vi "Send CALL.vi"(0 "WAMP Client in":refnum<class "WAMP Client.lvclass">, 5 "Call Request":T7, 9 "Message Loop Shift Register Data":T1, 11 "error in (no error)":errorcluster) -> (4 "WAMP Client out":refnum<class "WAMP Client.lvclass">, 10 "Message Loop Shift Register Data (out)":T1, 15 "error out":errorcluster)   [LabVIEW 2021, in "wamplv.lvlib" / "WAMP Client.lvclass"]
uses:
  WAMP Client.lvclass
  TypeDef/CALL Request Data.ctl
  API/TypeDefs/RESULT payload.ctl
  API/TypeDefs/Combined error.ctl
  API/TypeDefs/WAMP error.ctl
  TypeDef/Message Loop Shift Reg Data.ctl
  TypeDef/REGISTER Request Data.ctl
  TypeDef/Success or error.ctl
  TypeDef/Publish Requests Map.ctl
  TypeDef/PUBLISH Request Data.ctl
  TypeDef/PUBLISH result.ctl
  TypeDef/Endpoint Data.ctl
  TypeDef/CALL Request Map.ctl
  TypeDef/SUBSCRIBE Requests Map.ctl
  TypeDef/SUBSCRIBE Request Data.ctl
  TypeDef/Subscribe Result.ctl
  TypeDef/EVENT payload.ctl
  TypeDef/Subscriptions Map.ctl
  TypeDef/Subscription Details.ctl
  TypeDef/Unsubscribe Requests Map.ctl
  TypeDef/UNSUBSCRIBE Request Data.ctl
  TypeDef/UNSUBSCRIBE Result.ctl
  TypeDef/Unregister requests map.ctl
  TypeDef/Unregister request.ctl
  TypeDef/WAMP Message Codes.ctl
  WAMP Client.lvclass/WAMP Client.ctl
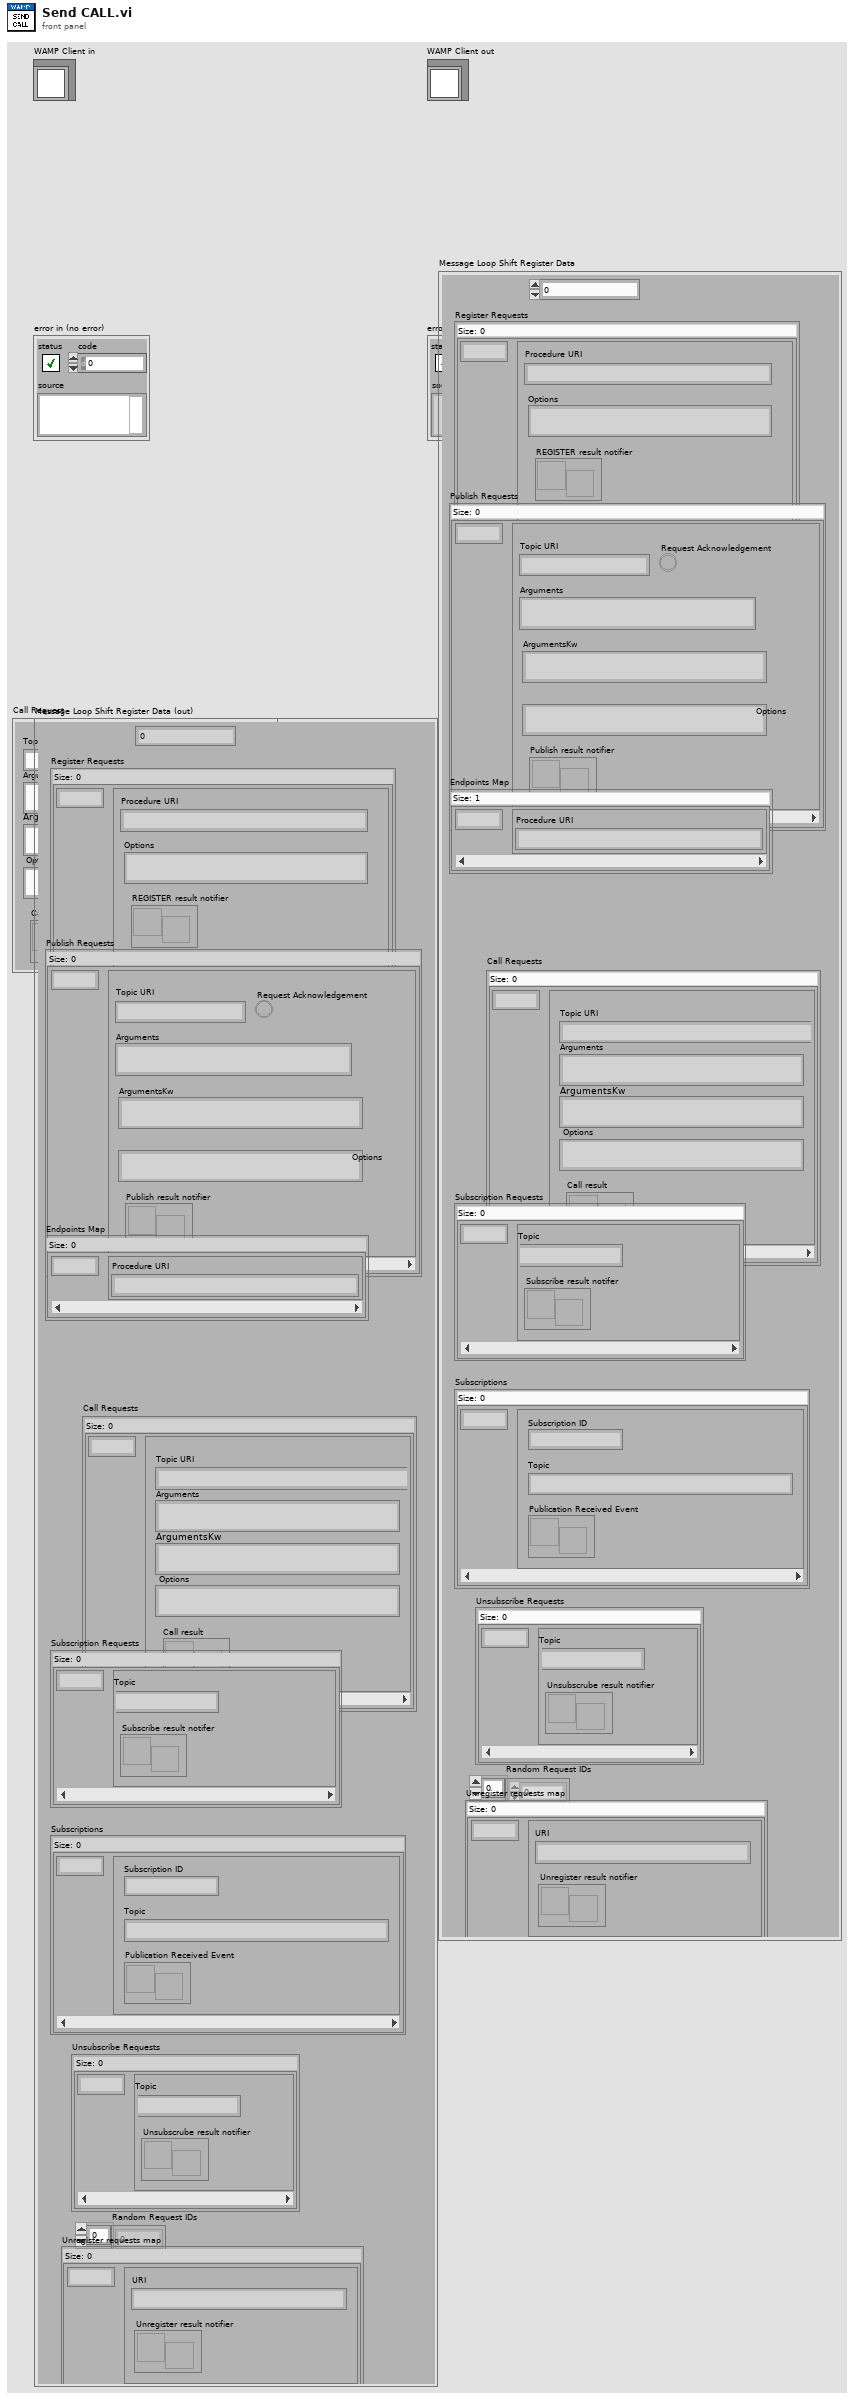
[diagram p1: front panel]
types:
  T1 = typedef "wamplv.lvlib/WAMP Client.lvclass/Message Loop Shift Reg Data.ctl" = cluster{"Last Request ID":u64, "Register Requests":map{u64, T2}, "Publish Requests":T3, "Endpoints Map":map{u64, T5}, "Call Requests":T6, "Subscription Requests":T8, "Subscriptions":T10, "Unsubscribe Requests":T12, "Random Request IDs":u64[], "Unregister requests map":T14}
  T2 = typedef "wamplv.lvlib/WAMP Client.lvclass/REGISTER Request Data.ctl" = cluster{"Procedure URI":string, "Options":string, "REGISTER result notifier":refnum<notifier>}
  T3 = typedef "wamplv.lvlib/WAMP Client.lvclass/Publish Requests Map.ctl" = map{u64, T4}
  T4 = typedef "wamplv.lvlib/WAMP Client.lvclass/PUBLISH Request Data.ctl" = cluster{"Topic URI":string, "Arguments":string, "ArgumentsKw":string, "Request Acknowledgement":bool, "Options":string, "Publish result notifier":refnum<notifier>}
  T5 = typedef "wamplv.lvlib/WAMP Client.lvclass/Endpoint Data.ctl" = cluster{"Procedure URI":string}
  T6 = typedef "wamplv.lvlib/WAMP Client.lvclass/CALL Request Map.ctl" = map{u64, T7}
  T7 = typedef "wamplv.lvlib/WAMP Client.lvclass/CALL Request Data.ctl" = cluster{"Topic URI":string, "Arguments":string, "ArgumentsKw":string, "Options":string, "Call result":refnum<notifier>}
  T8 = typedef "wamplv.lvlib/WAMP Client.lvclass/SUBSCRIBE Requests Map.ctl" = map{u64, T9}
  T9 = typedef "wamplv.lvlib/WAMP Client.lvclass/SUBSCRIBE Request Data.ctl" = cluster{"Topic":string, "Subscribe result notifer":refnum<notifier>}
  T10 = typedef "wamplv.lvlib/WAMP Client.lvclass/Subscriptions Map.ctl" = map{u64, T11}
  T11 = typedef "wamplv.lvlib/WAMP Client.lvclass/Subscription Details.ctl" = cluster{"Subscription ID":u64, "Topic":string, "Publication Received Event":refnum<user-event>}
  T12 = typedef "wamplv.lvlib/WAMP Client.lvclass/Unsubscribe Requests Map.ctl" = map{u64, T13}
  T13 = typedef "wamplv.lvlib/WAMP Client.lvclass/UNSUBSCRIBE Request Data.ctl" = cluster{"Topic":string, "Unsubscrube result notifier":refnum<notifier>}
  T14 = typedef "wamplv.lvlib/WAMP Client.lvclass/Unregister requests map.ctl" = map{u64, T15}
  T15 = typedef "wamplv.lvlib/WAMP Client.lvclass/Unregister request.ctl" = cluster{"URI":string, "Unregister result notifier":refnum<notifier>}
  T16 = typedef "wamplv.lvlib/WAMP Client.lvclass/WAMP Message Codes.ctl" = u16
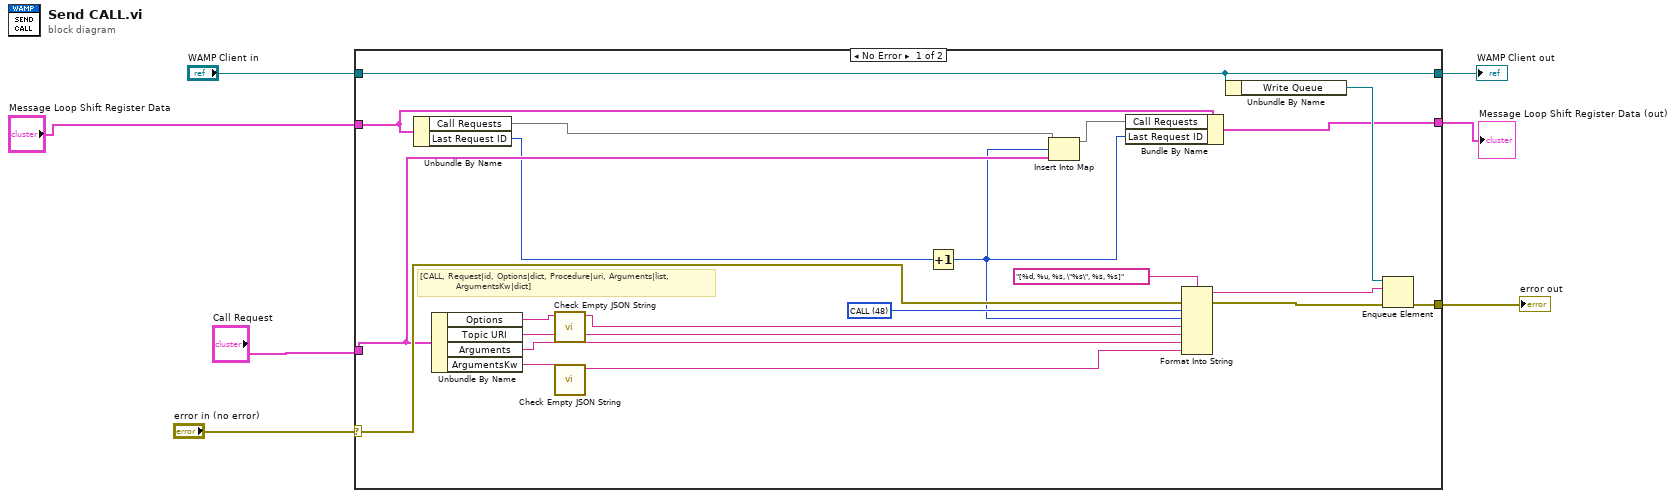
[diagram p0: block diagram]
diagram:
  n1 = case shown="No Error" "error in (no error)" {
    selector: "error in (no error)" -> [w23 w31]
    tunnel: [w28 w31] -> w6
    tunnel: [w22 w30] -> w4
    tunnel: "WAMP Client in" -> [w22 w30]
    tunnel: "Call Request" -> [w18 _]
    tunnel: "Message Loop Shift Register Data" -> [w15 w29]
    tunnel: [w14 w29] -> w1
    frame No Error {
      w20 = T16 48 items=["HELLO"=1, "WELCOME"=2, "ABORT"=3, "GOODBYE"=6, "ERROR"=8, "PUBLISH"=16, "PUBLISHED"=17, "SUBSCRIBE"=32, "SUBSCRIBED"=33, "UNSUBSCRIBE"=34, "UNSUBSCRIBED"=35, "EVENT"=36, "CALL"=48, "RESULT"=59, "REGISTER"=64, "REGISTERED"=65, "UNREGISTER"=66, "UNREGISTERED"=67, "INVOCATION"=68, "YIELD"=70] ("Message Codes")
      # "[CALL, Request|id, Options|dict, Procedure|uri, Arguments|list,\n            ArgumentsKw|dict]"
      n2 = Unbundle By Name(w15) -> ("Call Requests"=w17:T6, "Last Request ID"=w13:u64)
      n3 = Unbundle By Name(w18) -> ("Options"=w9:string, "Topic URI"=w19:string, "Arguments"=w21:string, "ArgumentsKw"=w11:string)
      n4 = call "Check Empty JSON String.vi"("JSON"=w9) -> ("JSON"=w8:string)  [unwired: 10 in]
      n5 = call "Check Empty JSON String.vi"("JSON"=w11) -> ("JSON"=w10:string)  [unwired: 10 in]
      n6 = Increment(x=w13) -> (x+1=w12:u64)
      n7 = Insert Into Map(map in=w17, key=w12, value=w18) -> (map out=w16:T6)  [unwired: 2 out]
      n8 = Bundle By Name(cluster=w15, "Call Requests"=w16, "Last Request ID"=w12) -> (w14:T1)
      n9 = Format Into String(format string="[%d, %u, %s, \"%s\", %s, %s]" ("element"), error in=w23, w20, w12, w8, w19, w21, w10) -> (resulting string=w26:string, error out=w25:errorcluster)  [unwired: 1 in]
      n10 = Unbundle By Name(w22) -> ("Write Queue"=w24:refnum<queue>)
      n11 = Enqueue Element(queue=w24, element=w26, error in (no error)=w25) -> (error out=w28:errorcluster)  [unwired: 1 in, 2 out]
    }
    frame Error {
    }
  }
  "error out" <- w6
  "WAMP Client out" <- w4
  "Message Loop Shift Register Data (out)" <- w1
